vi "Logging Message Loop.vi"(8 "error in (no error)":errorcluster, 10 "Data Queue":refnum<queue>, 11 "Message Queues":T1) -> (0 "error out":errorcluster)   [LabVIEW 2024, in "DAQ_msgHandler Logging.lvlib"]
doc: "The message loop subVI to handle messages pertaining to logging data."
uses:
  DAQ_msgHandler Logging.lvlib
  support/Message Queue/All Message Queues.ctl
  support/Message Queue/Message Cluster.ctl
  support/Message Queue/Enqueue Message (Single).vi
  <vilib>/Utility/error.llb/Error Cluster From Error Code.vi
  <vilib>/ErrorRing/Error Ring.xnode
  support/Message Queue/DAQ_msgHandler Message Queue.lvlib
  CTRsample/Control/streamIO_states.ctl
  controls/DAQ_msgHandler StreamTypeDef.ctl
panel:
  in  "Control Notifier":refnum<notifier>
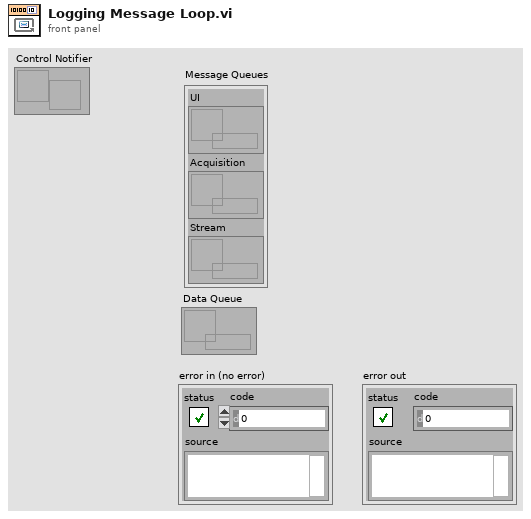
[diagram p1: front panel]
types:
  T1 = typedef "DAQ_msgHandler Message Queue.lvlib/All Message Queues.ctl" = cluster{"UI":refnum<queue>, "Acquisition":refnum<queue>, "Stream":refnum<queue>}
  T2 = typedef "streamIO_states.ctl" = enum16{"Fault", "Initilize", "Stream", "Close"}
  T3 = typedef "DAQ_msgHandler StreamTypeDef.ctl" = cluster{"stream state":T2, "DAQ Node":string, "DAQ Node ID":i32, "Writer Endpoint":refnum<k21>, "Reader Endpoint":refnum<k21>, "Stream Timeout":dbl, "Managment Timeout":dbl}
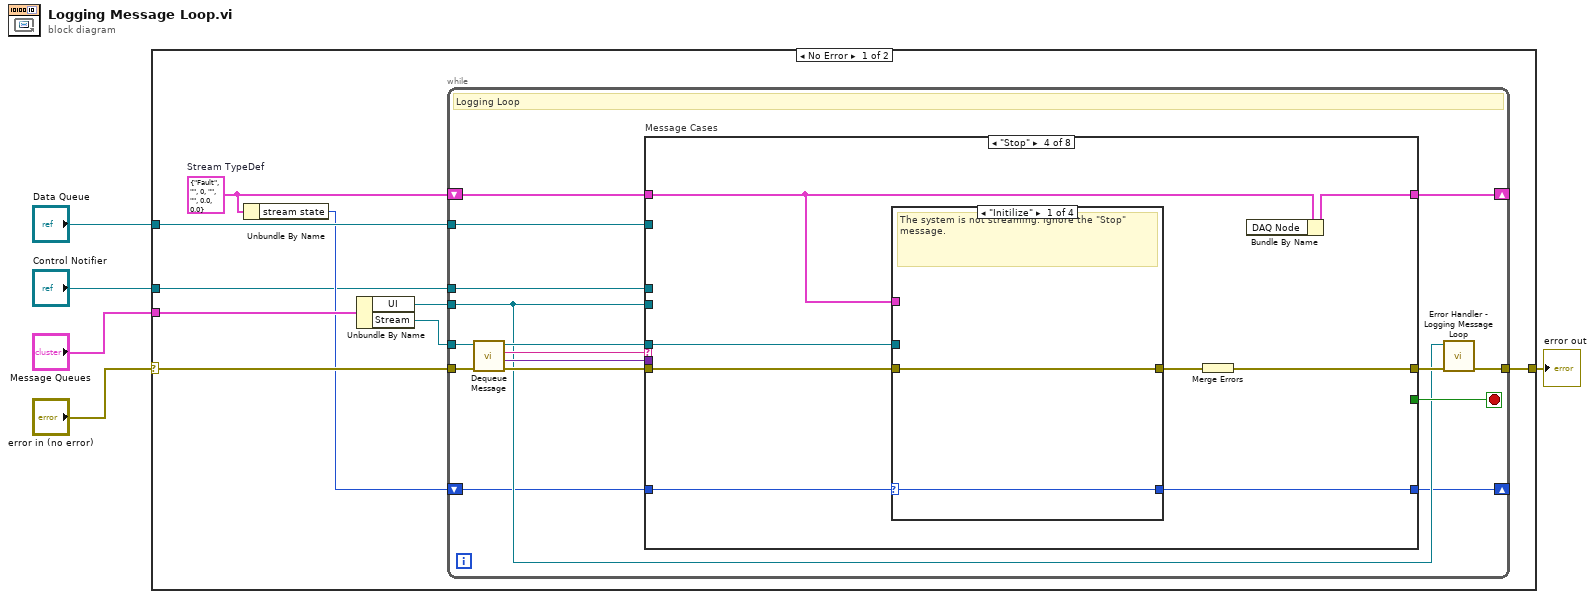
[diagram p0: block diagram]
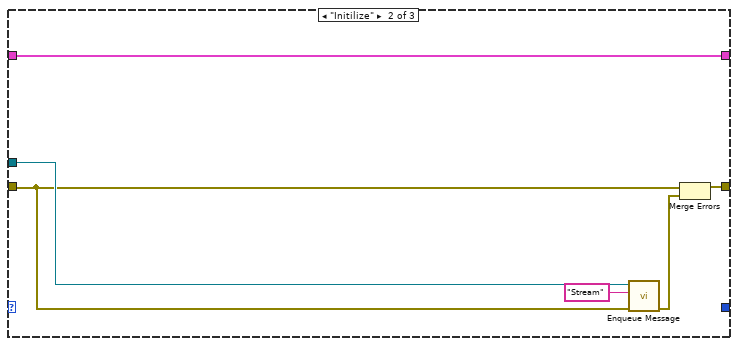
[diagram p5: hidden frame]
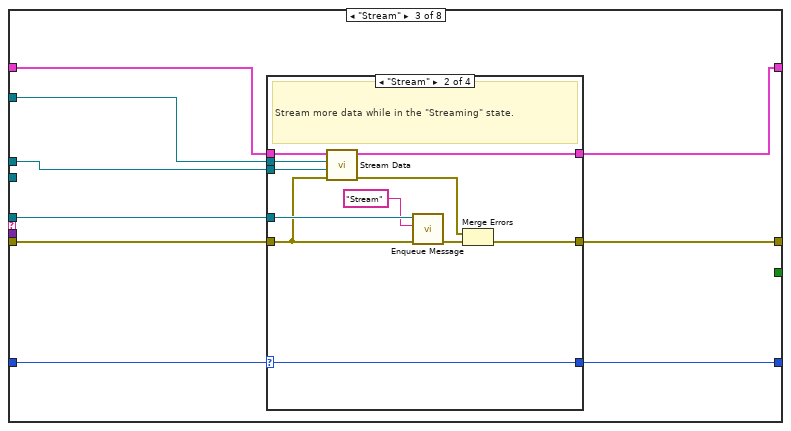
[diagram p6: hidden frame]
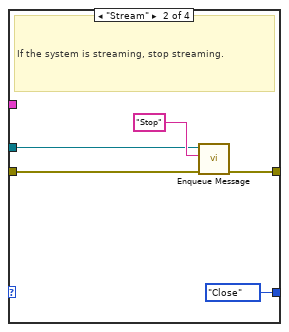
[diagram p10: hidden frame]
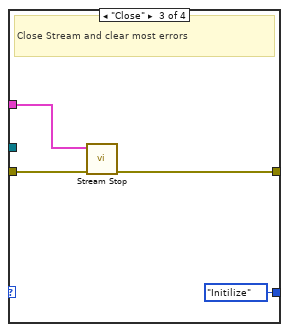
[diagram p11: hidden frame]
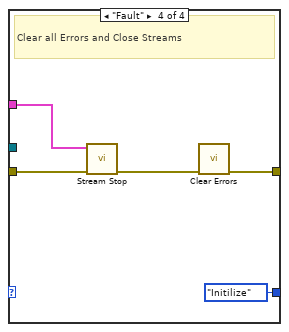
[diagram p12: hidden frame]
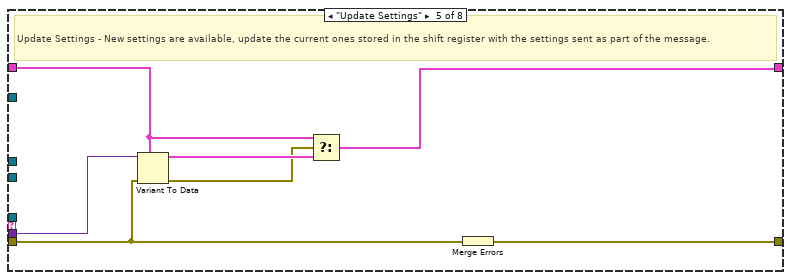
[diagram p13: hidden frame]
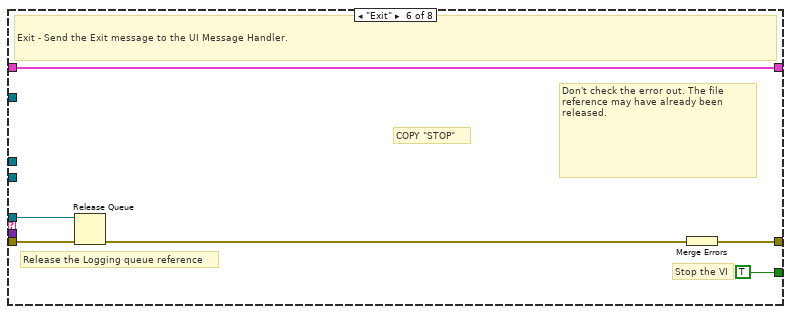
[diagram p14: hidden frame]
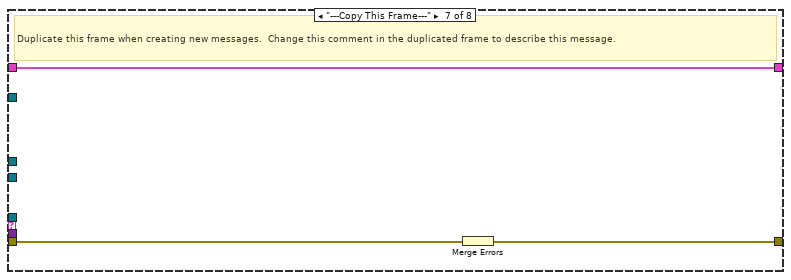
[diagram p15: hidden frame]
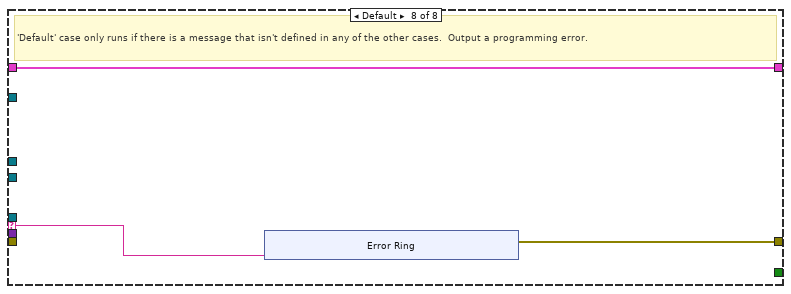
[diagram p16: hidden frame]
diagram:
  n1 = case shown="No Error" "error in (no error)" {
    selector: "error in (no error)" -> [w11 w129]
    tunnel: "Message Queues" -> [w14 _]
    tunnel: [w12 w129] -> w4
    tunnel: "Data Queue" -> [w10 _]
    tunnel: "Control Notifier" -> [w6 _]
    frame No Error {
      w8 = T3 {"stream state"=enum."Fault", "DAQ Node"="", "DAQ Node ID"=0, "Writer Endpoint"="", "Reader Endpoint"="", "Stream Timeout"=0.0, "Managment Timeout"=0.0}  # Stream TypeDef
      n2 = Unbundle By Name(w8) -> ("stream state"=w7:T2)
      n3 = Unbundle By Name(w14) -> ("UI"=w9:refnum<queue>, "Stream"=w13:refnum<queue>)
      n4 = while {
        tunnel: w13 -> [w22]
        shift-right: [w29] -> _
        shift-left: w8 -> [w30]
        tunnel: w9 -> [w18]
        tunnel: w10 -> [w21]
        tunnel: w11 -> [w27]
        tunnel: [w20] -> w12
        shift-right: [w16] -> _
        shift-left: w7 -> [w17]
        tunnel: w6 -> [w15]
        stop <- w28 stop-if-true
        # "Logging Loop"
        n5 = call "Dequeue Message.vi"("error in (no error)"=w27, "Message Queue"=w22) -> ("error out"=w26:errorcluster, "Message Data"=w24:variant, "Message"=w25:string, "dup Message Queue"=w23:refnum<queue>)  [unwired: 6 in]
        n6 = case "Message Cases" shown="\"Stop\"" w25 {
          selector: w25 -> [_ _ _ _ _ _ _ w119]
          tunnel: w23 -> [_ w38 w57 w79 _ w112 _ _]
          tunnel: w26 -> [w31 w37 w55 w82 w103 w113 w118 _]
          tunnel: [w31 w39 w58 w86 w109 w114 w116 w120] -> w19
          tunnel: w30 -> [w32 w36 w54 w83 w107 w110 w117 w121]
          tunnel: [w32 w35 w50 w84 w104 w110 w117 w121] -> w29
          tunnel: [_ _ _ _ _ TRUE _ _] -> w28
          tunnel: w24 -> [_ _ _ _ w108 _ _ _]
          tunnel: w18 -> [_ _ _ _ _ _ _ _]
          tunnel: w21 -> [_ _ w56 _ _ _ _ _]
          tunnel: w17 -> [_ w34 w53 w81 _ _ _ _]
          tunnel: [_ w33 w52 w80 _ _ _ _] -> w16
          tunnel: w15 -> [_ _ w51 _ _ _ _ _]
          frame "Initialize" {
            # "Initialize - gets called when first launched. Currently a no-op."
          }
          frame "Start" {
            n7 = case shown="\"Fault\"" w34 {
              selector: w34 -> [_ _ w48]
              tunnel: [w40 w44 w49] -> w39
              tunnel: w38 -> [_ w45 _]
              tunnel: w37 -> [w40 w43 w49]
              tunnel: w36 -> [w41 w42 _]
              tunnel: [w41 w42 _] -> w35
              tunnel: [_ _ w48] -> w33
              frame "Stream" {
                # "The system is already Streaming. Ignore the \"Start\" message."
              }
              frame "Initilize" {
                n8 = call-poly "Enqueue Message.vi"("error in (no error)"=w43, "Message"="Stream", "Message Queue"=w45) -> ("error out"=w46:errorcluster)  [unwired: 7 in, 1 out]
                n9 = Merge Errors(w43, w46) -> (w44:errorcluster)
              }
              frame "Fault" {
              }
            }
          }
          frame "Stream" {
            n10 = case shown="\"Stream\"" w53 {
              selector: w53 -> [w61 w66 w73 w76]
              tunnel: [w60 w72 w75 w78] -> w58
              tunnel: w57 -> [_ w70 _ _]
              tunnel: w56 -> [_ w69 _ _]
              tunnel: w55 -> [w60 w65 w75 w78]
              tunnel: w54 -> [w59 w64 w74 w77]
              tunnel: [w61 w66 w73 w76] -> w52
              tunnel: w51 -> [_ w63 _ _]
              tunnel: [w59 w62 w74 w77] -> w50
              frame "Initilize" {
                # "Ignore \"Stream\" messages when the streaming is idle."
              }
              frame "Stream" {
                # "Stream more data while in the \"Streaming\" state."
                n11 = call "Stream Data.vi"("error in (no error)"=w65, "Control Notifier"=w63, "Data Queue"=w69, "DAQ_msgHandler StreamTypeDef"=w64) -> ("error out"=w68:errorcluster, "DAQ_msgHandler StreamTypeDef 2"=w62:T3)  [unwired: 6 in]
                n12 = call-poly "Enqueue Message.vi"("error in (no error)"=w65, "Message"="Stream", "Message Queue"=w70) -> ("error out"=w71:errorcluster)  [unwired: 7 in, 1 out]
                n13 = Merge Errors(w68, w71) -> (w72:errorcluster)
              }
              frame "Close" {
              }
              frame "Fault" {
              }
            }
          }
          frame "Stop" {
            n14 = case shown="\"Initilize\"" w81 {
              selector: w81 -> [w87 _ _ _]
              tunnel: [w88 w90 w94 w98] -> w85
              tunnel: w83 -> [_ _ w96 w101]
              tunnel: w82 -> [w88 w91 w95 w100]
              tunnel: [w87 streamIO_states."Close" ("stream state") streamIO_states."Initilize" ("stream state") streamIO_states."Initilize" ("stream state")] -> w80
              tunnel: w79 -> [_ w89 _ _]
              frame "Initilize" {
                # "The system is not streaming. Ignore the \"Stop\" message."
              }
              frame "Stream" {
                # "If the system is streaming, stop streaming."
                n15 = call-poly "Enqueue Message.vi"("error in (no error)"=w91, "Message"="Stop", "Message Queue"=w89) -> ("error out"=w90:errorcluster)  [unwired: 7 in, 1 out]
              }
              frame "Close" {
                # "Close Stream and clear most errors"
                n16 = call "Stream Stop.vi"("error in (no error)"=w95, "DAQ_msgHandler StreamTypeDef"=w96) -> ("error out"=w94:errorcluster)  [unwired: 8 in, 1 out]
              }
              frame "Fault" {
                # "Clear all Errors and Close Streams"
                n17 = call "Stream Stop.vi"("error in (no error)"=w100, "DAQ_msgHandler StreamTypeDef"=w101) -> ("error out"=w99:errorcluster)  [unwired: 8 in, 1 out]
                n18 = call <vilib>:"Clear Errors.vi"("error in (no error)"=w99) -> ("error out"=w98:errorcluster)  [unwired: 5 in, 1 out]
              }
            }
            n19 = Merge Errors(w85) -> (w86:errorcluster)
            n20 = Bundle By Name(cluster=w83) -> (w84:T3)  [unwired: 1 in]
          }
          frame "Update Settings" {
            # "Update Settings - New settings are available, update the current ones stored in the shift register with the settings sent as part of the message."
            n21 = Variant To Data(error in=w103, type=w107, Variant=w108) -> (data=w106:T3, error out=w105:errorcluster)
            n22 = Select(t=w107, s=w105, f=w106) -> (s? t:f=w104:T3)
            n23 = Merge Errors(w103) -> (w109:errorcluster)
          }
          frame "Exit" {
            # "COPY \"STOP\""
            # "Don't check the error out. The file reference may have already been released."
            # "Release the Logging queue reference"
            # "Stop the VI"
            # "Exit - Send the Exit message to the UI Message Handler."
            n24 = Release Queue(queue=w112, error in (no error)=w113) -> (error out=w111:errorcluster)  [unwired: 1 in, 2 out]
            n25 = Merge Errors(w111) -> (w114:errorcluster)
          }
          frame "---Copy This Frame---" {
            # "Duplicate this frame when creating new messages.  Change this comment in the duplicated frame to describe this message."
            n26 = Merge Errors(w118) -> (w116:errorcluster)
          }
          frame Default {
            # "'Default' case only runs if there is a message that isn't defined in any of the other cases.  Output a programming error."
            n27 = xnode "Error Ring"("parameter 0"=w119) -> ("error out"=w120:errorcluster)
          }
        }
        n28 = call "Error Handler - Logging Message Loop.vi"("error in (no error)"=w19, "Message Queue"=w18) -> ("dup error in"=w20:errorcluster)  [unwired: 8 in, 1 out]
      }
    }
    frame Error {
    }
  }
  "error out" <- w4
